vi "Updater Split Prompted Input Files.vi"(8 "error in (no error)":errorcluster, 11 "source file path (*.tdms)":path) -> (0 "error out":errorcluster, 3 "source file path (*.tdms) out":path)   [LabVIEW 2011]
doc: "Converts the specified file from the .tdms file format to the .tdm file format."
panel:
  out "group names":string[](array[string])
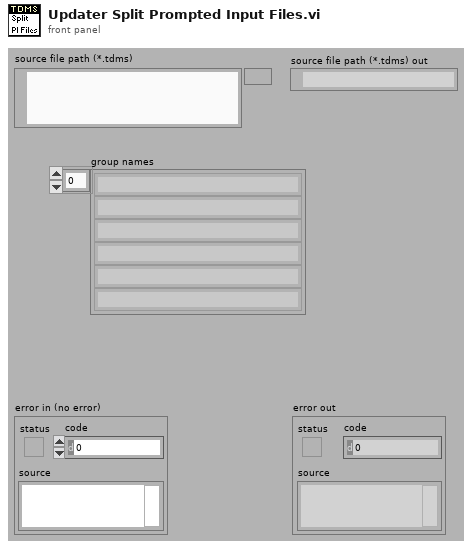
[diagram p1: front panel]
types:
  T1 = enum16{"open", "open or create", "create or replace", "create", "open (read-only)"}
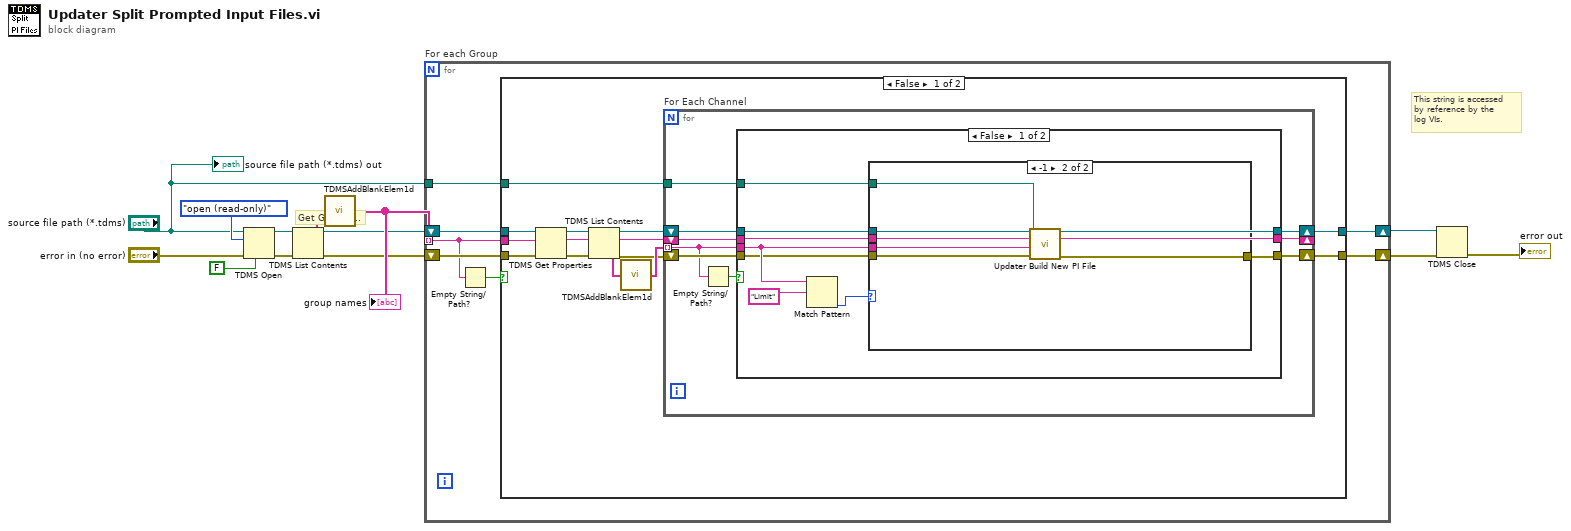
[diagram p0: block diagram]
diagram:
  # "Get Groups..."
  # "This string is accessed\nby reference by the\nlog VIs."
  n1 = TDMS Open(6:FALSE ("disable buffering (T)"), 8:"error in (no error)", 10:T1."open (read-only)" ("TDMS File Operation"), 11:"source file path (*.tdms)") -> (0:w13:errorcluster, 3:w12:refnum<k34>)  [unwired: 2 in]
  n2 = TDMS List Contents(4:w13, 7:w12) -> (0:w5:errorcluster, 2:w1:string[], 3:w9:refnum<k34>)  [unwired: 2 out]
  n3 = call <vilib>:"TDMSAddBlankElem1d.vi"("input string array"=w1) -> ("output string array with blank element at the beginning"=w10:string[])
  "group names" <- w10
  n4 = for "For each Group" {
    shift-right: [w19] -> w8
    shift-left: w9 -> [w20]
    tunnel: w10 -> [w15] mode=indexing
    shift-right: [w18] -> w6
    shift-left: w5 -> [w17]
    tunnel: "source file path (*.tdms)" -> [w14]
    n5 = Empty String/Path?(string/path=w15) -> (empty?=w16:bool)
    n6 = case shown="False" w16 {
      tunnel: w20 -> [w34 w61]
      tunnel: [w28 w61] -> w19
      tunnel: w15 -> [w27 _]
      tunnel: [w26 w62] -> w18
      tunnel: w17 -> [w25 w62]
      tunnel: w14 -> [w22 _]
      frame False {
        n7 = TDMS Get Properties(8:w25, 10:w27, 11:w34) -> (0:w24:errorcluster, 2:w32:string, 3:w33:refnum<k34>)  [unwired: 6 out]
        n8 = TDMS List Contents(4:w24, 6:w32, 7:w33) -> (0:w23:errorcluster, 1:w21:string[], 2:w31:string, 3:w29:refnum<k34>)
        n9 = call <vilib>:"TDMSAddBlankElem1d.vi"("input string array"=w21) -> ("output string array with blank element at the beginning"=w30:string[])
        n10 = for "For Each Channel" {
          tunnel: w30 -> [w36] mode=indexing
          shift-right: [w40] -> _
          shift-left: w31 -> [w42]
          shift-right: [w41] -> w28
          shift-left: w29 -> [w43]
          shift-right: [w39] -> w26
          shift-left: w23 -> [w38]
          tunnel: w22 -> [w35]
          n11 = Empty String/Path?(string/path=w36) -> (empty?=w37:bool)
          n12 = case shown="False" w37 {
            tunnel: w43 -> [w48 w60]
            tunnel: w42 -> [w46 w59]
            tunnel: [w48 w60] -> w41
            tunnel: [w46 w59] -> w40
            tunnel: [w45 w58] -> w39
            tunnel: w38 -> [w47 w58]
            tunnel: w36 -> [w51 _]
            tunnel: w35 -> [w44 _]
            frame False {
              n13 = Match Pattern(string=w51, regular expression="Limit") -> (offset past match=w49:i32)  [unwired: 4 out]
              n14 = case shown="-1" w49 {
                tunnel: w51 -> [_ w53]
                tunnel: w48 -> [_ _]
                tunnel: w47 -> [w52 w57]
                tunnel: w46 -> [_ w54]
                tunnel: [w52 w56] -> w45
                tunnel: w44 -> [_ w55]
                frame Default {
                }
                frame -1 {
                  n15 = call "Updater Build New PI File.vi"("error in (no error)"=w57, "Channel Name"=w53, "Source Run ID"=w54, "Source File"=w55) -> ("error out"=w56:errorcluster)  [unwired: 7 out]
                }
              }
            }
            frame True {
            }
          }
        }
      }
      frame True {
      }
    }
  }
  n16 = TDMS Close(8:w6, 11:w8) -> (0:→"error out":errorcluster)  [unwired: 1 out]
  "source file path (*.tdms) out" <- "source file path (*.tdms)"
